vi "Draw Panel into Subpanel Procedure.vi"(8 "error in":errorcluster, 10 "SubPanel in":refnum<vi>, 11 "This VI":refnum<vi>) -> (0 "error out":errorcluster, 3 "SubPanel out":refnum<vi>)   [LabVIEW 2020, in "Monochromator.lvlib"]
doc: "____\nPantherLAB Templates 1.0.0.5\nCopyright (c) 2022, PantherLAB"
uses:
  Monochromator.lvlib
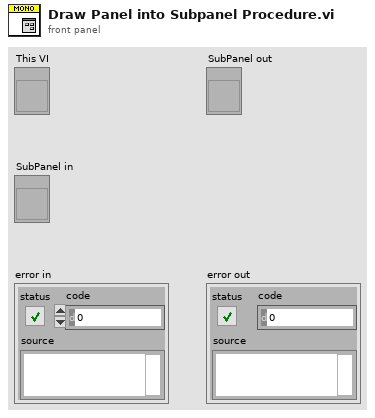
[diagram p1: front panel]
types:
  T1 = enum32{"Invalid", "Standard", "Closed", "Hidden", "Minimized", "Maximized"}
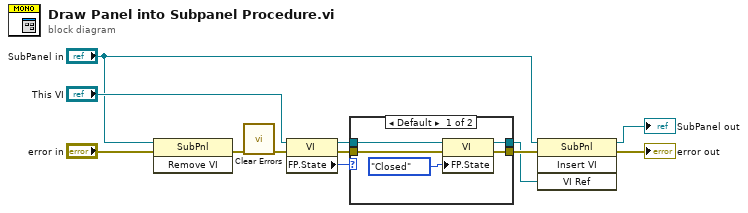
[diagram p0: block diagram]
diagram:
  n1 = invoke class="SubPnl" method="Remove VI"(reference="SubPanel in", error in="error in") -> (error out=w11:errorcluster)  [unwired: 1 in, 2 out]
  n2 = call <vilib>:"Clear Errors.vi"("error in (no error)"=w11) -> ("error out"=w12:errorcluster)  [unwired: 5 in, 1 out]
  n3 = property class="VI"(reference="This VI", error in=w12) -> (reference out=w4:refnum<vi>, error out=w10:errorcluster, "FP.State"=w6:T1)
  n4 = case shown="Default" w6 {
    tunnel: w4 -> [w15 w18]
    tunnel: w10 -> [w17 w19]
    tunnel: [w16 w19] -> w9
    tunnel: [w13 w18] -> w2
    frame Default {
      n5 = property class="VI"(reference=w15, error in=w17, "FP.State"=T1."Closed" ("Front Panel Window:State")) -> (reference out=w13:refnum<vi>, error out=w16:errorcluster)
    }
    frame "Closed" {
    }
  }
  n6 = invoke class="SubPnl" method="Insert VI"(reference="SubPanel in", error in=w9, "VI Ref"=w2) -> (reference out=→"SubPanel out":refnum<vi>, error out=→"error out":errorcluster)  [unwired: 1 in, 2 out]
